vi "automatic_step_finish.vi"(7 "transition_queue":refnum<queue>, 8 "error in (no error)":errorcluster, 10 "data":variant, 11 "recipe_data":variant) -> (0 "error out":errorcluster)   [LabVIEW 2015, in "lv-recipe-machine.lvlib" / "example_02.lvlib"]
uses:
  example_02.lvlib
  public/_controls/transition.ctl
  lv-recipe-machine.lvlib
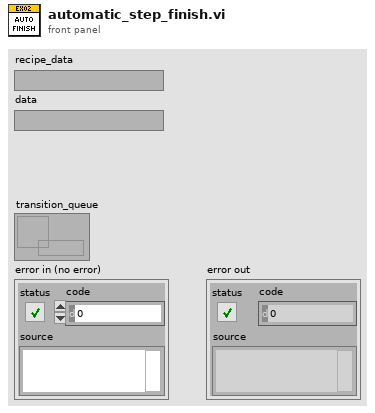
[diagram p1: front panel]
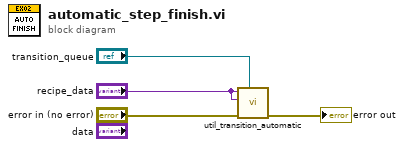
[diagram p0: block diagram]
diagram:
  n1 = call "util_transition_automatic.vi"("transition_queue"="transition_queue", "error in (no error)"="error in (no error)", "data"="recipe_data", "recipe_data"="recipe_data") -> ("error out"=→"error out":errorcluster)  [unwired: 7 in]
